vi "motor-position-query-v2-k1.vi"(8 "error in (no error)":errorcluster, 10 "Unit":enum16{"fs", "ps", "um", "mm", "counts"}(ring), 11 "Axis Select":u8(slide)=1 min=1 max=4 scale=1.0..4.0) -> (0 "error out":errorcluster, 1 "Initial Position of motor":string, 2 "Initial Position in selected unit":dbl, 3 "Initial Position in counts":dbl)   [LabVIEW 2009]
doc: "This VI provides the current position of PI stage in selected unit as well as the machine language counts and a string for position with unit."
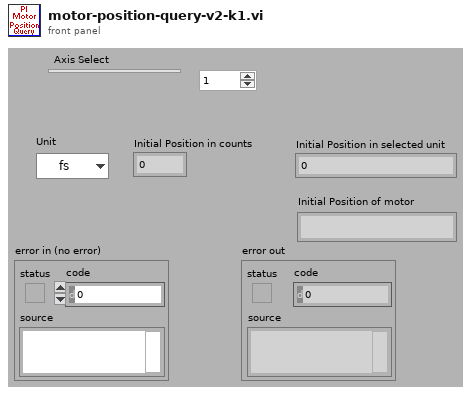
[diagram p1: front panel]
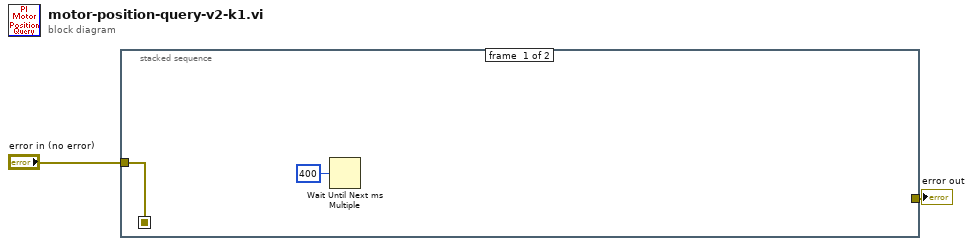
[diagram p0: block diagram]
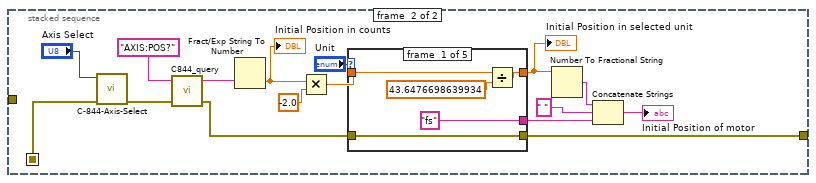
[diagram p2: hidden frame]
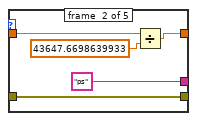
[diagram p3: hidden frame]
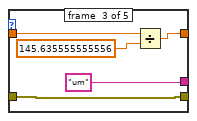
[diagram p4: hidden frame]
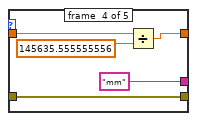
[diagram p5: hidden frame]
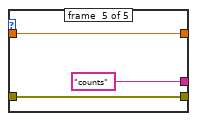
[diagram p6: hidden frame]
diagram:
  n1 = stacked-sequence {
    seq-local: [w3 _] -> [_ w8]
    tunnel: "error in (no error)" -> [w3 _]
    tunnel: [_ w5] -> w1
    frame #0 {
      n2 = Wait Until Next ms Multiple(millisecond multiple=u32 400) -> ()  [unwired: 1 out]
    }
    frame #1 {
      n3 = call "C-844-Axis-Select.vi"("error in (no error)"=w8, "Axis Select"="Axis Select") -> ("error out"=w10:errorcluster)  [unwired: 8 in, 1 out]
      n4 = call "C844_query.vi"("Error in"=w10, "Command"="AXIS:POS?") -> ("Error out"=w6:errorcluster, "Response"=w20:string)  [unwired: 2 in]
      n5 = Fract/Exp String To Number(string=w20) -> (number=w13:dbl)  [unwired: 3 in, 1 out]
      "Initial Position in counts" <- w13
      n6 = Multiply(x=w13, y=-2.0) -> (x*y=w11:dbl)
      n7 = case shown="\"um\"" "Unit" {
        tunnel: w11 -> [w24 w29 w34 w39 w43]
        tunnel: [w23 w28 w33 w38 w43] -> w14
        tunnel: ["fs" "ps" "um" "mm" "counts"] -> w7
        tunnel: w6 -> [w21 w26 w31 w36 w41]
        tunnel: [w21 w26 w31 w36 w41] -> w5
        frame #0 {
          n8 = Divide(x=w24, y=43.6476698639934) -> (x/y=w23:dbl)
        }
        frame #1 {
          n9 = Divide(x=w29, y=43647.6698639933) -> (x/y=w28:dbl)
        }
        frame #2 {
          n10 = Divide(x=w34, y=145.635555555556) -> (x/y=w33:dbl)
        }
        frame #3 {
          n11 = Divide(x=w39, y=145635.555555556) -> (x/y=w38:dbl)
        }
        frame #4 {
        }
      }
      "Initial Position in selected unit" <- w14
      n12 = Number To Fractional String(number=w14) -> (F-format string=w18:string)  [unwired: 3 in]
      n13 = Concatenate Strings(w18, " ", w7) -> (→"Initial Position of motor":string)
    }
  }
  "error out" <- w1
